vi "Read Assertion Parameters.vi"(8 "error in (no error)":errorcluster, 10 "Schema Version":string, 11 "refnum":T5) -> (0 "error out":errorcluster, 2 "Macro Step":T1={"Type"=enum."Mouse Move", "X"=0, "Y"=0, "Delay"=0, "Key"=65, "Repeat"=0, "RClick?"=FALSE, "App/Window Name"="", "Notes"="", "Assertion Type"=enum."Control Position", "Control Name"="", "Disabled"=enum."Enabled", "Visible"=enum."Visible", "Left"=0, "Top"=0, "Width"=0, "Height"=0, "Expected Image"={"image type"=0, "image depth"=0, "image"=[], "mask"=[], "colors"=[], "Rectangle"={"left"=0, "top"=0, "right"=0, "bottom"=0}}}, 3 "refnum out":T5)   [LabVIEW 2020, in "MacroAssert.lvlib"]
doc: "Reads the list of steps from macro config file defined by <B>refnum</B>."
uses:
  MacroAssert.lvlib
  <vilib>/Utility/config.llb/NI_LVConfig.lvlib
  CTLs/Step Type V3.ctl
  CTLs/Step V3.ctl
  <vilib>/ErrorRing/Error Ring.xnode
  <vilib>/Utility/config.llb/Read Key (String).vi
  CTLs/Assertion Type.ctl
  <vilib>/Utility/config.llb/Read Key (Boolean).vi
  <vilib>/Utility/config.llb/Read Key (U32).vi
  <vilib>/picture/picture.llb/imagedata.ctl
  <vilib>/Utility/error.llb/Error Cluster From Error Code.vi
  <vilib>/Utility/config.llb/Config Data RefNum.ctl
panel:
  in  "Section":string
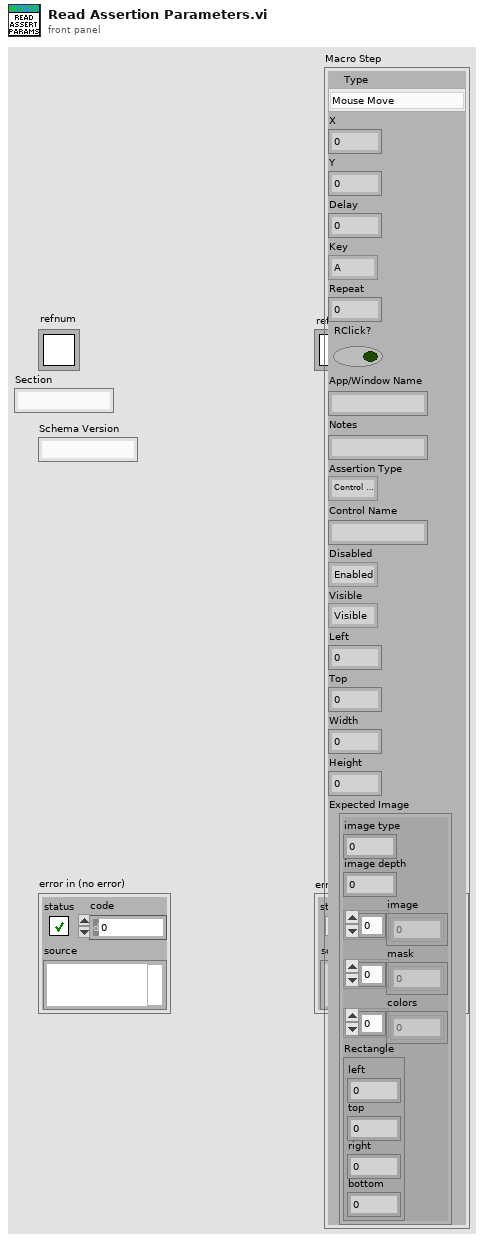
[diagram p1: front panel]
types:
  T1 = typedef "MacroAssert.lvlib/Step V3.ctl" = cluster{"Type":T2, "X":i32, "Y":i32, "Delay":i32, "Key":u8, "Repeat":i32, "RClick?":bool, "App/Window Name":string, "Notes":string, "Assertion Type":T3, "Control Name":string, "Disabled":enum8{"Enabled", "Disabled", "Disabled and Grayed Out"}, "Visible":enum16{"Visible", "Not Visible"}, "Left":i16, "Top":i16, "Width":i16, "Height":i16, "Expected Image":T4}
  T2 = typedef "MacroAssert.lvlib/Step Type V3.ctl" = enum16{"Mouse Move", "Mouse Click", "Key Press", "Wait", "Mouse Down", "Mouse Up", "Key Down", "Key Up", "Test Assertion", "Run Application", "Maximize Window", "Restore Window", "Minimize Window", "Close Window", "Bring Window to Front", "Send Window to Back"}
  T3 = typedef "MacroAssert.lvlib/Assertion Type.ctl" = enum16{"Control Position", "Control Visible", "Control Disabled", "Control Image"}
  T4 = typedef "imagedata.ctl" = cluster{"image type":i32, "image depth":i32, "image":u8[], "mask":u8[], "colors":u32[], "Rectangle":cluster{"left":i16, "top":i16, "right":i16, "bottom":i16}}
  T5 = typedef "NI_LVConfig.lvlib/Config Data RefNum.ctl" = refnum<k1>
  T6 = enum8{"Enabled", "Disabled", "Disabled and Grayed Out"}
  T7 = cluster{"value":string, enum8{"Enabled", "Disabled", "Disabled and Grayed Out"}}
  T8 = cluster{"value":string, cluster{"[0]":i32, "[1]":i32}}
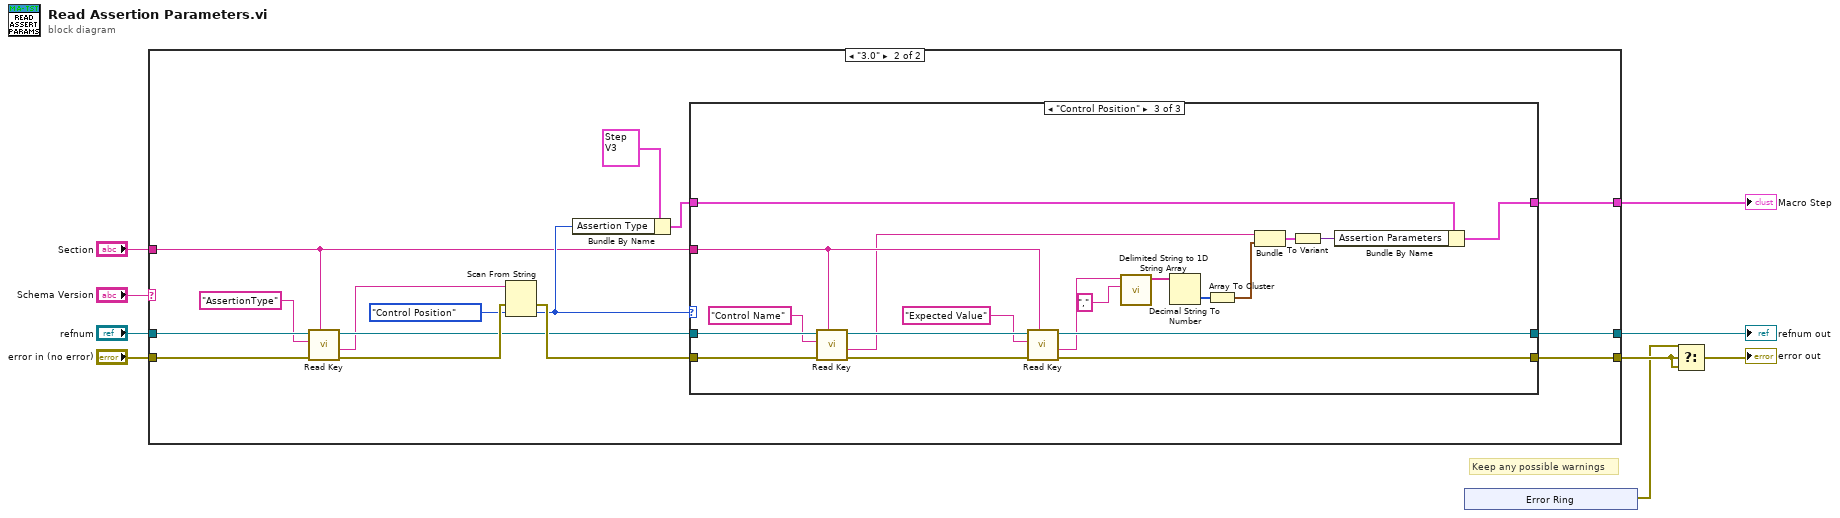
[diagram p0: block diagram]
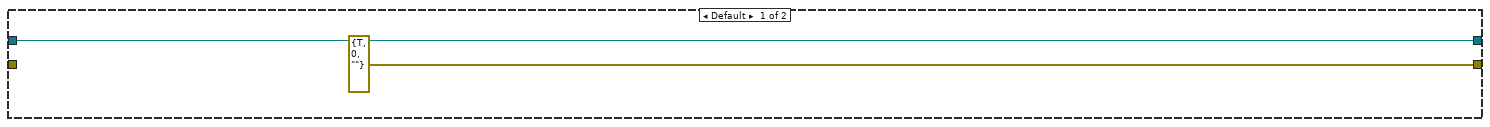
[diagram p2: hidden frame]
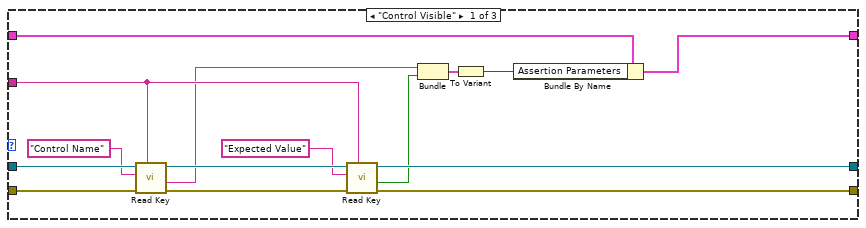
[diagram p3: hidden frame]
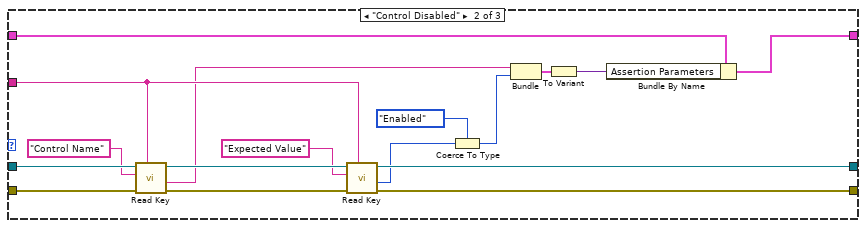
[diagram p4: hidden frame]
diagram:
  # "Keep any possible warnings"
  n1 = case shown="\"3.0\"" "Schema Version" {
    tunnel: "refnum" -> [w11 w23]
    tunnel: [w11 w25] -> w3
    tunnel: [errorcluster {"status"=TRUE, "code"=0, "source"=""} ("error out") w26] -> w9
    tunnel: "error in (no error)" -> [_ w24]
    tunnel: [_ w22] -> w2
    tunnel: "Section" -> [_ w12]
    frame Default {
    }
    frame "3.0" {
      n2 = call-poly <vilib>:"Read Key.vi"("section"=w12, "error in (no error)"=w24, "key"="AssertionType", "refnum"=w23) -> ("error out"=w20:errorcluster, "value"=w16:string, "refnum out"=w17:T5)  [unwired: 4 in, 1 out]
      n3 = Scan From String(input string=w16, error in=w20, default 1=Assertion_Type."Control Position" ("Assertion Type")) -> (error out=w21:errorcluster, output 1=w14:T3)  [unwired: 2 in, 2 out]
      n4 = Bundle By Name(cluster=T1 {"Type"=enum."Mouse Move", "X"=0, "Y"=0, "Delay"=0, "Key"=65, "Repeat"=0, "RClick?"=FALSE, "App/Window Name"="", "Notes"="", "Assertion Type"=enum."Control Position", "Control Name"="", "Disabled"=enum."Enabled", "Visible"=enum."Visible", "Left"=0, "Top"=0, "Width"=0, "Height"=0, "Expected Image"={"image type"=0, "image depth"=0, "image"=[], "mask"=[], "colors"=[], "Rectangle"={"left"=0, "top"=0, "right"=0, "bottom"=0}}} ("Step"), "Assertion Type"=w14) -> (w13:T1)
      n5 = case shown="\"Control Position\"" w14 {
        tunnel: w21 -> [w40 w57 w76]
        tunnel: w17 -> [w39 w56 w75]
        tunnel: w12 -> [w33 w50 w69]
        tunnel: [w35 w52 w71] -> w26
        tunnel: [w34 w51 w70] -> w25
        tunnel: [w27 w45 w64] -> w22
        tunnel: w13 -> [w29 w47 w66]
        frame "Control Visible" {
          n6 = call-poly <vilib>:"Read Key.vi"("section"=w33, "error in (no error)"=w40, "key"="Control Name", "refnum"=w39) -> ("error out"=w36:errorcluster, "value"=w31:string, "refnum out"=w41:T5)  [unwired: 4 in, 1 out]
          n7 = call-poly <vilib>:"Read Key.vi"("section"=w33, "error in (no error)"=w36, "key"="Expected Value", "refnum"=w41) -> ("error out"=w35:errorcluster, "value"=w32:bool, "refnum out"=w34:T5)  [unwired: 4 in, 1 out]
          n8 = Bundle("value"=w31, "value"=w32) -> (w30:cluster{"value":string, "value":bool})  [unwired: 1 in]
          n9 = To Variant(anything=w30) -> (Variant=w28:variant)
          n10 = Bundle By Name(cluster=w29, "Assertion Parameters"=w28) -> (w27:T1)
        }
        frame "Control Disabled" {
          n11 = call-poly <vilib>:"Read Key.vi"("section"=w50, "error in (no error)"=w57, "key"="Control Name", "refnum"=w56) -> ("error out"=w53:errorcluster, "value"=w49:string, "refnum out"=w58:T5)  [unwired: 4 in, 1 out]
          n12 = call-poly <vilib>:"Read Key.vi"("section"=w50, "error in (no error)"=w53, "key"="Expected Value", "refnum"=w58) -> ("error out"=w52:errorcluster, "value"=w43:u32, "refnum out"=w51:T5)  [unwired: 4 in, 1 out]
          n13 = Coerce To Type(0:w43, 1:T6."Enabled") -> (2:w42:T6)
          n14 = Bundle("value"=w49, w42) -> (w48:T7)  [unwired: 1 in]
          n15 = To Variant(anything=w48) -> (Variant=w46:variant)
          n16 = Bundle By Name(cluster=w47, "Assertion Parameters"=w46) -> (w45:T1)
        }
        frame "Control Position" {
          n17 = call-poly <vilib>:"Read Key.vi"("section"=w69, "error in (no error)"=w76, "key"="Control Name", "refnum"=w75) -> ("error out"=w72:errorcluster, "value"=w68:string, "refnum out"=w77:T5)  [unwired: 4 in, 1 out]
          n18 = call-poly <vilib>:"Read Key.vi"("section"=w69, "error in (no error)"=w72, "key"="Expected Value", "refnum"=w77) -> ("error out"=w71:errorcluster, "value"=w63:string, "refnum out"=w70:T5)  [unwired: 4 in, 1 out]
          n19 = call <vilib>:"Delimited String to 1D String Array.vi"("delimiter"=",", "delimited string"=w63) -> ("string array"=w61:string[])  [unwired: 9 in]
          n20 = Decimal String To Number(string=w61) -> (number=w60:i32[])  [unwired: 2 in, 1 out]
          n21 = Array To Cluster(array=w60) -> (cluster=w59:cluster{"[0]":i32, "[1]":i32})
          n22 = Bundle("value"=w68, w59) -> (w67:T8)  [unwired: 1 in]
          n23 = To Variant(anything=w67) -> (Variant=w65:variant)
          n24 = Bundle By Name(cluster=w66, "Assertion Parameters"=w65) -> (w64:T1)
        }
      }
    }
  }
  "refnum out" <- w3
  "Macro Step" <- w2
  n25 = xnode "Error Ring"() -> ("error out"=w8:errorcluster)
  n26 = Select(t=w8, s=w9, f=w9) -> (s? t:f=→"error out":errorcluster)
